vi "Switch Shutdown (7001).vi"(8 "error in (no error)":errorcluster, 11 "VISA resource name in":refnum<visa-resource-name>) -> (0 "error out":errorcluster, 3 "VISA resource name out":refnum<visa-resource-name>)   [LabVIEW 2016, in "Hall Effect Library.lvlib"]
uses:
  Hall Effect Library.lvlib
  <instrlib>/Keithley 7001/Keithley 7001.lvlib
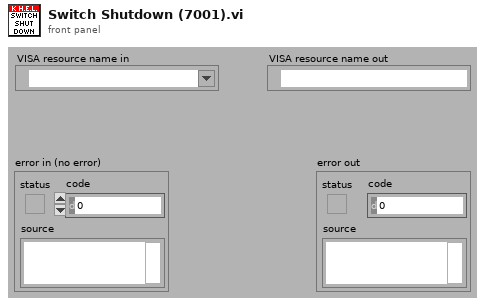
[diagram p1: front panel]
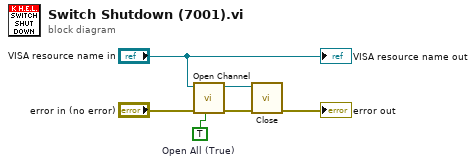
[diagram p0: block diagram]
diagram:
  w3 = TRUE  # Open All (True)
  n1 = call <instrlib>:"Open Channel.vi"("Open All (False)"=w3, "error in (no error)"="error in (no error)", "VISA resource name"="VISA resource name in") -> ("error out"=w6:errorcluster, "VISA resource name out"=w5:refnum<visa-resource-name>)  [unwired: 1 in, 6 out]
  n2 = call <instrlib>:"Close.vi"("error in (no error)"=w6, "VISA resource name"=w5) -> ("error out"=→"error out":errorcluster)  [unwired: 9 out]
  "VISA resource name out" <- "VISA resource name in"
